vi "VersionCheck.vi"(4 "error in (no error)":errorcluster, 6 "Version":string) -> (0 "error out":errorcluster, 2 "outdated?":bool, 3 "Latest Version":string)   [LabVIEW 2024]
uses:
  <vilib>/regexp/Match Regular Expression.xnode
panel:
  out "standard output":string
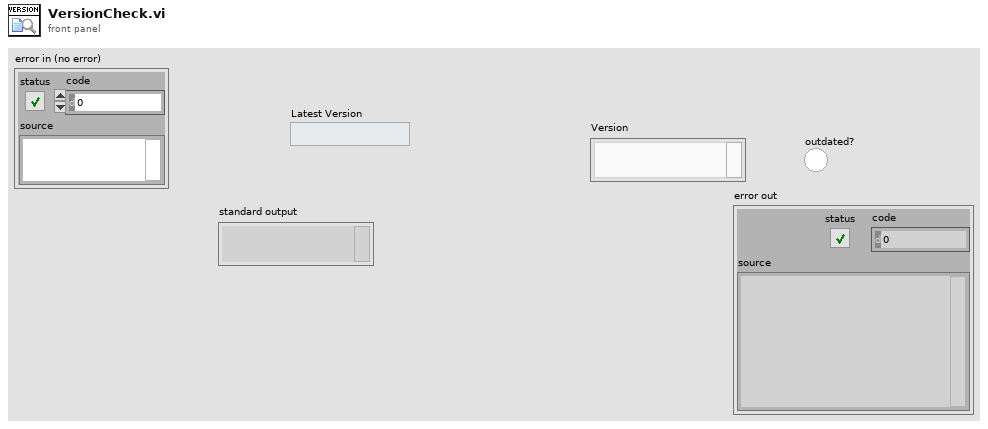
[diagram p1: front panel]
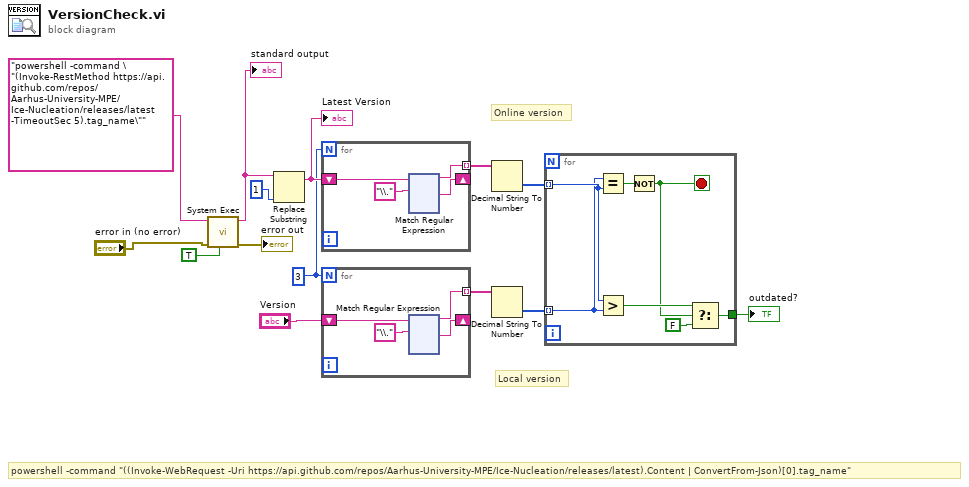
[diagram p0: block diagram]
diagram:
  w1 = 3
  # "Local version"
  # "Online version"
  # "powershell -command \"((Invoke-WebRequest -Uri https://api.github.com/repos/Aarhus-University-MPE/Ice-Nucleation/releases/latest).Content | ConvertFrom-Json)[0].tag_name\""
  n1 = call <vilib>:"System Exec.vi"("run minimized? (F)"=TRUE, "error in (no error)"="error in (no error)", "command line"="powershell -command \"(Invoke-RestMethod https://api.github.com/repos/Aarhus-University-MPE/Ice-Nucleation/releases/latest -TimeoutSec 5).tag_name\"") -> ("error out"=→"error out":errorcluster, "standard output"=w8:string)  [unwired: 5 in, 2 out]
  "standard output" <- w8
  n2 = Replace Substring(2:1 ("length (len. of substring)"), 5:w8) -> (1:w6:string)  [unwired: 2 in, 1 out]
  "Latest Version" <- w6
  n3 = for {
    N: w1 -> [_]
    shift-right: [w16] -> _
    shift-left: w6 -> [w17]
    tunnel: [w15] -> w5 mode=indexing
    n4 = xnode "Match Regular Expression"("input string"=w17, "regular expression"="\\.") -> ("before match"=w15:string, "after match"=w16:string)  [unwired: 4 in, 3 out]
  }
  n5 = for {
    N: w1 -> [_]
    shift-right: [w137] -> _
    shift-left: "Version" -> [w138]
    tunnel: [w136] -> w3 mode=indexing
    n6 = xnode "Match Regular Expression"("input string"=w138, "regular expression"="\\.") -> ("before match"=w136:string, "after match"=w137:string)  [unwired: 4 in, 3 out]
  }
  n7 = Decimal String To Number(string=w5) -> (number=w4:i32[])  [unwired: 2 in, 1 out]
  n8 = Decimal String To Number(string=w3) -> (number=w2:i32[])  [unwired: 2 in, 1 out]
  n9 = for {
    tunnel: w4 -> [w262] mode=indexing
    tunnel: w2 -> [w261] mode=indexing
    tunnel: [w258] -> w14
    stop <- w257 stop-if-true
    n10 = Equal?(x=w261, y=w262) -> (x = y?=w263:bool)
    n11 = Greater?(x=w262, y=w261) -> (0:w260:bool)
    n12 = Not(x=w263) -> (.not. x?=w257:bool)
    n13 = Select(t=w260, s=w257, f=FALSE) -> (s? t:f=w258:bool)
  }
  "outdated?" <- w14
